vi "temp.vi"() -> ()   [LabVIEW 2021]
uses:
  <vilib>/DAQmx/read.llb/DAQmx Read (Analog DBL 1Chan 1Samp).vi
  <vilib>/DAQmx/create/channels.llb/DAQmx Create Channel (AI-Temperature-Thermocouple).vi
  <vilib>/DAQmx/miscellaneous.llb/DAQmx Fill In Error Info.vi
panel:
  out "Waveform Chart":dbl(graph)
  out "TEMP":dbl format="%0.2f"
  in  "physical channels":tag
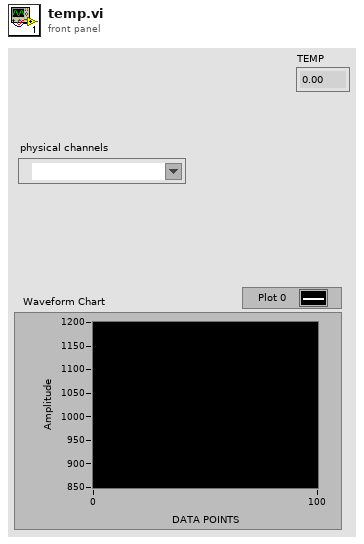
[diagram p1: front panel]
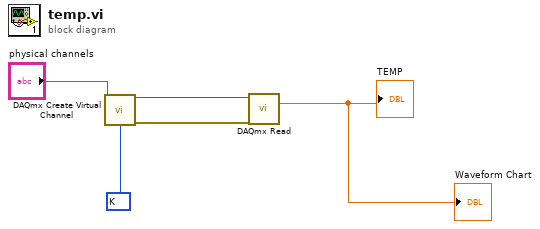
[diagram p0: block diagram]
diagram:
  w4 = 10073 items=["J"=10072, "K"=10073, "N"=10077, "R"=10082, "S"=10085, "T"=10086, "B"=10047, "E"=10055] ("thermocouple type")
  n1 = call-poly <vilib>:"DAQmx Create Virtual Channel.vi"("physical channels"="physical channels", "thermocouple type"=w4) -> ("task out"=w3:refnum<k21>, "error out"=w2:errorcluster)  [unwired: 12 in]
  n2 = call-poly <vilib>:"DAQmx Read.vi"("task/channels in"=w3, "error in"=w2) -> ("data"=→"TEMP" →"Waveform Chart":dbl)  [unwired: 11 in, 2 out]
